vi "PID_scalar (derivative acts only on process variable).vi"(5 "T_d":dbl=1.0, 7 "T_i":dbl=1.0, 9 "process variable":dbl, 10 "set point":dbl, 11 "K_p":dbl=1.0) -> (2 "output":dbl)   [LabVIEW 2011]
uses:
  <vilib>/Simulation/Implementation/Shared/SIMSCR Execution Mode.ctl
  <vilib>/Simulation/Scripting/Companion Diagram/SimConfigNode/SimParams.ctl
  <vilib>/Simulation/Scripting/Companion Diagram/SimConfigNode/_simSolvers.ctl
  <vilib>/Simulation/Param Hierarchy/Typedefs/SIMPH Param Control Actions.ctl
  <vilib>/Simulation/Implementation/Shared/SIM limit type.ctl
  <vilib>/Simulation/ContinuousLinear/Implementation/NILVSim Derivative.llb/SIM derivative (scalar).vi
  <vilib>/Simulation/SignalArithmetic/Implementation/NILVSim Gain.llb/SIM Gain (scalar).vi
  <vilib>/Simulation/ContinuousLinear/Implementation/NILVSim Integrator new.llb/SIM Integrator distributor (scalar).vi
  <vilib>/Simulation/ContinuousLinear/Implementation/NILVSim Integrator new.llb/SIM Integrator collector (scalar).vi
  <vilib>/Simulation/Implementation/Shared/NILVSim_Manager.vi
  <vilib>/Simulation/Implementation/Shared/NILVSim_ParamChanged.vi
  <vilib>/Simulation/Implementation/Shared/NILVSim_FinalizeModel.vi
  <vilib>/Simulation/Implementation/Shared/SIM Unbundle Sim Info.vi
  <vilib>/Simulation/Implementation/Shared/NILVSim_GetModelError.vi
  <vilib>/Simulation/Implementation/Shared/SIM SimErrorHandler.vi
  <vilib>/Simulation/Implementation/Shared/SIM Bundle Sim Info.vi
  <vilib>/Simulation/Implementation/Shared/NILVSim_Initialize.vi
  <vilib>/Simulation/Scripting/Companion Diagram/SimConfigNode/SimDog.xnode
  <vilib>/Simulation/Implementation/XNodeFramework/SimXNode/SimX.xnode
  <vilib>/Simulation/ContinuousLinear/Implementation/NILVSim Integrator new.llb/SIM Integrator (scalar).vi
  <vilib>/Simulation/Implementation/Shared/NI_SIM_Implementation.lvlib
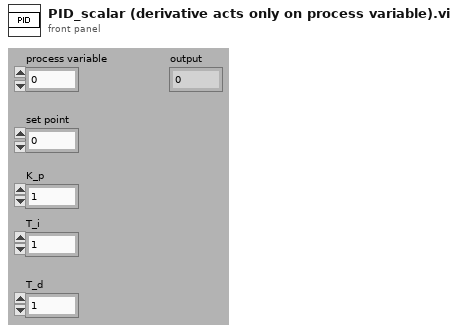
[diagram p1: front panel]
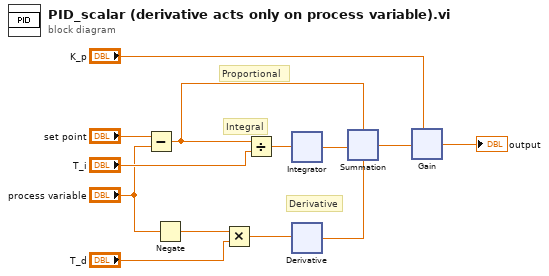
[diagram p0: block diagram]
diagram:
  # "Derivative"
  # "Integral"
  # "Proportional"
  n1 = Subtract(x="set point", y="process variable") -> (x-y=w6:dbl)
  n2 = Negate(x="process variable") -> (-x=w4:dbl)
  n3 = Multiply(x=w4, y="T_d") -> (x*y=w2:dbl)
  n4 = Divide(x=w6, y="T_i") -> (x/y=w13:dbl)
  n5 = xnode ("Integrator")("input"=w13) -> ("output"=w11:dbl)  [unwired: 9 in, 2 out]
  n6 = xnode ("Derivative")("input"=w2) -> ("output"=w1:dbl)  [unwired: 2 in]
  n7 = xnode ("Summation")("Operand1"=w6, "Operand2"=w11, "Operand3"=w1) -> ("Result"=w10:dbl)
  n8 = xnode ("Gain")("gain"="K_p", "input"=w10) -> ("output"=→"output":dbl)  [unwired: 2 in]
